vi "ForLoop-Ver1.vi"() -> ()   [LabVIEW 2018]
panel:
  out "For Loop Count":string
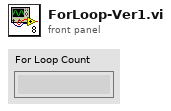
[diagram p1: front panel]
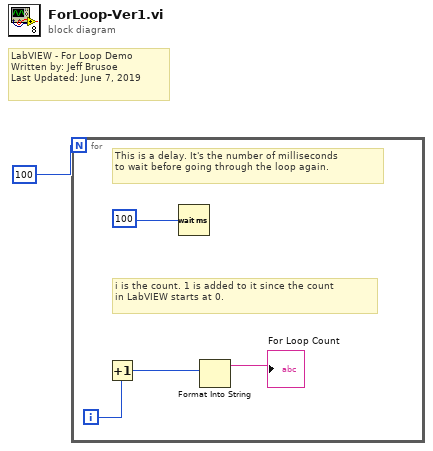
[diagram p0: block diagram]
diagram:
  # "LabVIEW - For Loop Demo\nWritten by: Jeff Brusoe\nLast Updated: June 7, 2019"
  n1 = for {
    N: 100 -> [_]
    i -> [w3]
    # "i is the count. 1 is added to it since the count\nin LabVIEW starts at 0."
    # "This is a delay. It's the number of milliseconds\nto wait before going through the loop again."
    n2 = Increment(x=w3) -> (x+1=w2:i32)
    n3 = Wait (ms)(milliseconds to wait=u32 100 ("millisecond timer value")) -> ()  [unwired: 1 out]
    n4 = Format Into String(w2) -> (resulting string=→"For Loop Count":string)  [unwired: 3 in, 1 out]
  }
